vi "lib LV Timestamp to SCLK.vi"(8 "error in (no error)":errorcluster, 11 "lv timestamp in":timestamp format="%<%H:%M:%S%3u\n%x>T") -> (0 "error out":errorcluster, 3 "SCLK":dbl format="%#_11f")   [LabVIEW 2015]
panel:
  in  "J2000 Epoch":timestamp=timestamp(3029590736 s since 1904-01-01) format="%<%H:%M:%S%2u\n%x>T"
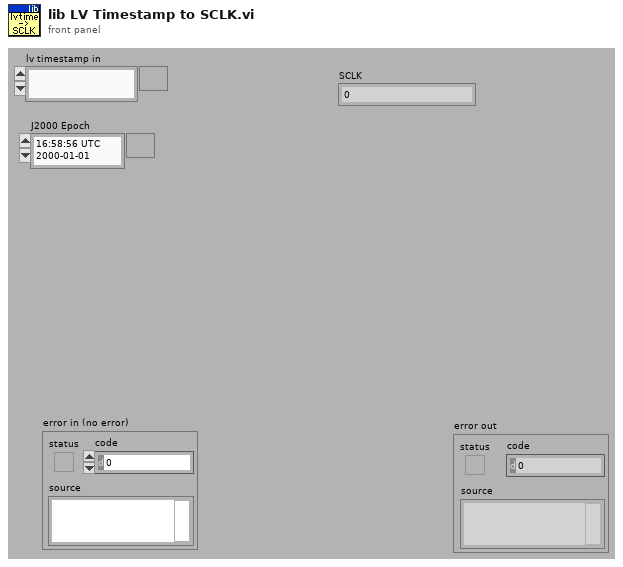
[diagram p1: front panel]
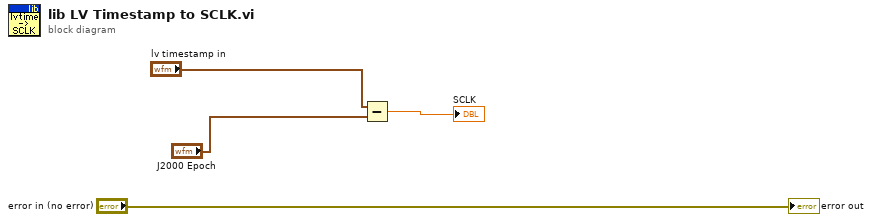
[diagram p0: block diagram]
diagram:
  n1 = Subtract(x="lv timestamp in", y="J2000 Epoch") -> (x-y=→"SCLK":dbl)
  "error out" <- "error in (no error)"
